vi "Add Records.vi"(7 "Bulk Insert?":bool, 8 "Error In (no error)":errorcluster, 10 "Expenses Tracker Records In":refnum<class "Expenses Tracker Record.lvclass">[](array[class]), 11 "SQLite DB Operator In":refnum<class "SQLite DB Operator.lvclass">) -> (0 "Error Out":errorcluster, 2 "Expenses Tracker Records Out":refnum<class "Expenses Tracker Record.lvclass">[](array[class]), 3 "SQLite DB Operator Out":refnum<class "SQLite DB Operator.lvclass">)   [LabVIEW 2023, in "SQLite DB Operator.lvclass"]
uses:
  SQLite DB Operator.lvclass
  Interfaces/Expenses Tracker Record/Expenses Tracker Record.lvclass
  SQLite DB Operator.lvclass/SQLite DB Operator.ctl
  <vilib>/drjdpowell/SQLite Library/SQL Statement/SQL Statement.lvclass/SQL Statement.ctl
  <vilib>/drjdpowell/SQLite Library/SQL Statement/Step.vi
  Private/VIs/Prepare Insert Row Command.vi
  Private/VIs/Bind Insert Command Parameters.vi
  <vilib>/drjdpowell/SQLite Library/SQL Statement/Error Message.vi
  <vilib>/drjdpowell/SQLite Library/SQL Connection/Connection.lvclass
  <vilib>/drjdpowell/SQLite Library/SQL Statement/SQL Statement.lvclass
  <vilib>/drjdpowell/SQLite Library/Transaction Helpers/Transaction.lvlib
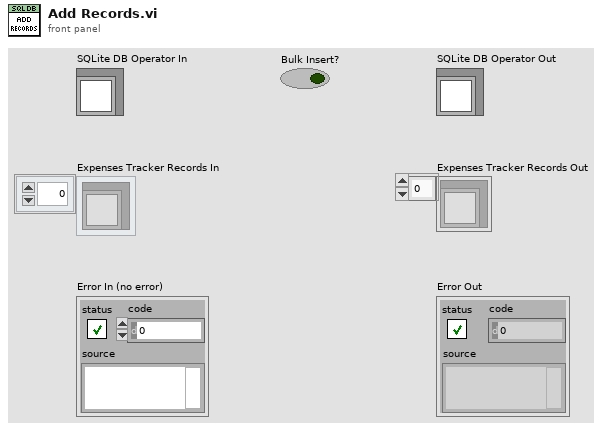
[diagram p1: front panel]
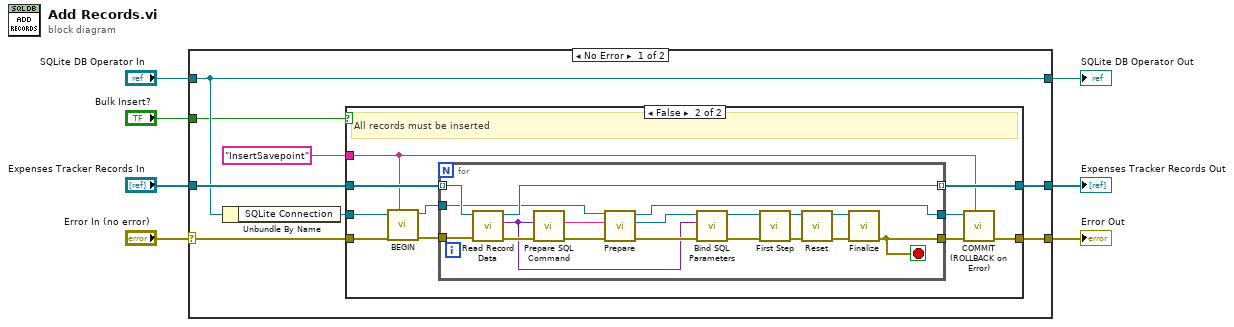
[diagram p0: block diagram]
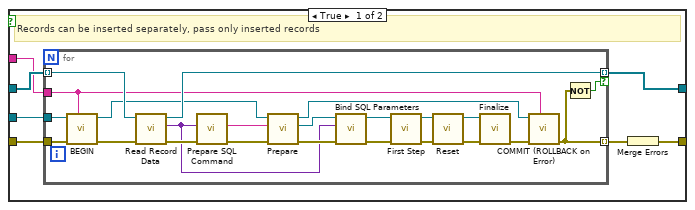
[diagram p2: hidden frame]
diagram:
  n1 = case shown="No Error" "Error In (no error)" {
    selector: "Error In (no error)" -> [w13 w76]
    tunnel: [w11 w76] -> w5
    tunnel: [w14 w75] -> w7
    tunnel: "SQLite DB Operator In" -> [w14 w75]
    tunnel: "Expenses Tracker Records In" -> [w15 w74]
    tunnel: [w10 w74] -> w2
    tunnel: "Bulk Insert?" -> [w8 _]
    frame No Error {
      n2 = Unbundle By Name(w14) -> ("SQLite Connection"=w12:refnum<class "Connection.lvclass">)
      n3 = case shown="False" w8 {
        tunnel: w15 -> [w22 w55]
        tunnel: w13 -> [w21 w52]
        tunnel: w12 -> [w20 w51]
        tunnel: [w16 w46] -> w11
        tunnel: [w18 w54] -> w10
        tunnel: "InsertSavepoint" ("Savepoint name") -> [w17 w53]
        frame True {
          # "Records can be inserted separately, pass only inserted records"
          n4 = for {
            tunnel: w21 -> [w31]
            tunnel: w22 -> [w33] mode=indexing
            tunnel: [w23] -> w19 mode=indexing
            tunnel: [w32] -> w18 mode=indexing if=w26
            tunnel: w17 -> [w27]
            tunnel: w20 -> [w29]
            n5 = call <vilib>:"BEGIN.vi"("Savepoint name"=w27, "error in (no error)"=w31, "SQLite Connection in"=w29) -> ("error out"=w30:errorcluster, "SQLite Connection"=w28:refnum<class "Connection.lvclass">)  [unwired: 7 in]
            n6 = call-dynamic "Read Record Data.vi"("Error In (no error)"=w30, "Expenses Tracker Record In"=w33) -> ("Error Out"=w41:errorcluster, "Record"=w35:variant, "Expenses Tracker Record Out"=w32:refnum<class "Expenses Tracker Record.lvclass">)  [unwired: 7 in]
            n7 = call-poly "Prepare SQL Command.vi"("Error In (no error)"=w41, "Record"=w35) -> ("Error Out"=w37:errorcluster, "Insert SQL Command"=w34:string)  [unwired: 8 in]
            n8 = call <vilib>:"Prepare.vi"("error in (no error)"=w37, "SQL"=w34, "SQLite Connection in"=w28) -> ("error out"=w36:errorcluster, "SQL Statement"=w38:refnum<class "SQL Statement.lvclass">, "SQLite Connection"=w24:refnum<class "Connection.lvclass">)  [unwired: 4 in, 2 out]
            n9 = call-poly "Bind SQL Parameters.vi"("Error In (no error)"=w36, "Record"=w35, "SQL Statement In"=w38) -> ("Error Out"=w39:errorcluster, "SQL Statement Out"=w40:refnum<class "SQL Statement.lvclass">)  [unwired: 7 in]
            n10 = call <vilib>:"First Step.vi"("error in (no error)"=w39, "SQL Statement in"=w40) -> ("error out"=w43:errorcluster, "SQL Statement"=w42:refnum<class "SQL Statement.lvclass">)  [unwired: 7 in, 1 out]
            n11 = call <vilib>:"Reset.vi"("error in (no error)"=w43, "SQL Statement in"=w42) -> ("error out"=w45:errorcluster, "SQL Statement"=w44:refnum<class "SQL Statement.lvclass">)  [unwired: 8 in]
            n12 = call <vilib>:"Finalize.vi"("error in (no error)"=w45, "SQL Statement in"=w44) -> ("error out"=w25:errorcluster)  [unwired: 9 in]
            n13 = call <vilib>:"COMMIT (ROLLBACK on Error).vi"("Savepoint name"=w27, "error in (no error)"=w25, "SQLite Connection in"=w24) -> ("error out"=w23:errorcluster)  [unwired: 7 in, 1 out]
            n14 = Not(x=w23) -> (.not. x?=w26:bool)
          }
          n15 = Merge Errors(w19) -> (w16:errorcluster)
        }
        frame False {
          # "All records must be inserted"
          n16 = call <vilib>:"BEGIN.vi"("Savepoint name"=w53, "error in (no error)"=w52, "SQLite Connection in"=w51) -> ("error out"=w50:errorcluster, "SQLite Connection"=w49:refnum<class "Connection.lvclass">)  [unwired: 7 in]
          n17 = for {
            tunnel: w55 -> [w61] mode=indexing
            tunnel: [w60] -> w54 mode=indexing
            tunnel: w50 -> [w59]
            tunnel: w49 -> [w58]
            tunnel: [w56] -> w48
            tunnel: [w57] -> w47
            stop <- w56 stop-if-true
            n18 = call-dynamic "Read Record Data.vi"("Error In (no error)"=w59, "Expenses Tracker Record In"=w61) -> ("Error Out"=w69:errorcluster, "Record"=w63:variant, "Expenses Tracker Record Out"=w60:refnum<class "Expenses Tracker Record.lvclass">)  [unwired: 7 in]
            n19 = call-poly "Prepare SQL Command.vi"("Error In (no error)"=w69, "Record"=w63) -> ("Error Out"=w65:errorcluster, "Insert SQL Command"=w62:string)  [unwired: 8 in]
            n20 = call <vilib>:"Prepare.vi"("error in (no error)"=w65, "SQL"=w62, "SQLite Connection in"=w58) -> ("error out"=w64:errorcluster, "SQL Statement"=w66:refnum<class "SQL Statement.lvclass">, "SQLite Connection"=w57:refnum<class "Connection.lvclass">)  [unwired: 4 in, 2 out]
            n21 = call-poly "Bind SQL Parameters.vi"("Error In (no error)"=w64, "Record"=w63, "SQL Statement In"=w66) -> ("Error Out"=w67:errorcluster, "SQL Statement Out"=w68:refnum<class "SQL Statement.lvclass">)  [unwired: 7 in]
            n22 = call <vilib>:"First Step.vi"("error in (no error)"=w67, "SQL Statement in"=w68) -> ("error out"=w71:errorcluster, "SQL Statement"=w70:refnum<class "SQL Statement.lvclass">)  [unwired: 7 in, 1 out]
            n23 = call <vilib>:"Reset.vi"("error in (no error)"=w71, "SQL Statement in"=w70) -> ("error out"=w73:errorcluster, "SQL Statement"=w72:refnum<class "SQL Statement.lvclass">)  [unwired: 8 in]
            n24 = call <vilib>:"Finalize.vi"("error in (no error)"=w73, "SQL Statement in"=w72) -> ("error out"=w56:errorcluster)  [unwired: 9 in]
          }
          n25 = call <vilib>:"COMMIT (ROLLBACK on Error).vi"("Savepoint name"=w53, "error in (no error)"=w48, "SQLite Connection in"=w47) -> ("error out"=w46:errorcluster)  [unwired: 7 in, 1 out]
        }
      }
    }
    frame Error {
    }
  }
  "Error Out" <- w5
  "SQLite DB Operator Out" <- w7
  "Expenses Tracker Records Out" <- w2
